vi "GroveSensors.vi"() -> ()   [LabVIEW 2016]
uses:
  VIs/uPythonX/uPythonX.xctl
panel:
  in  "Tab Control":enum32{"Button", "Pot", "Numbers"}(tab)=enum."Numbers"
  in  "Button":T1(xcontrol)={"VISA Refnum in"="ASRL23::INSTR", "Python Code"="import pyb,utime\n\nbutton = pyb.Pin('W16')\n\nbutton()\nutime.sleep(10)\nbutton()\n"}
  in  "Button 2":T1(xcontrol)={"VISA Refnum in"="ASRL23::INSTR", "Python Code"="import pyb,utime\n\nadc = pyb.ADC('W24')\n\nwhile True:\n     val = adc.read()\n     print ('%4.2f' % val)\n     utime.sleep_ms(200)\n     "}
  in  "Button 3":T1(xcontrol)={"VISA Refnum in"="ASRL23::INSTR", "Python Code"="import utime\n\ncharmap = {\n    '0': 0x3f,\n    '1': 0x06,\n    '2': 0x5b,\n    '3': 0x4f,\n    '4': 0x66,\n    '5': 0x6d,\n    '6': 0x7d,\n    '7': 0x07,\n    '8': 0x7f,\n    '9': 0x6f,\n    'A': 0x77,\n    'B': 0x7f,\n    'b': 0x7C,\n    'C': 0x39,\n    'c': 0x58,\n    'D': 0x3f,\n    'd': 0x5E,\n    'E': 0x79,\n    'F': 0x71,\n    'G': 0x7d,\n    'H': 0x76,\n    'h': 0x74,\n    'I': 0x06,\n    'J': 0x1f,\n    'K': 0x76,\n    'L': 0x38,\n    'l': 0x06,\n    'n': 0x54,\n    'O': 0x3f,\n    'o': 0x5c,\n    'P': 0x73,\n    'r': 0x50,\n    'S': 0x6d,\n    'U': 0x3e,\n    'V': 0x3e,\n    'Y': 0x66,\n    'Z': 0x5b,\n    '-': 0x40,\n    '_': 0x08,\n    ' ': 0x00\n}\n\nADDR_AUTO = 0x40\nADDR_FIXED = 0x44\nSTARTADDR = 0xC0\nBRIGHT_DARKEST = 0\nBRIGHT_DEFAULT = 2\nBRIGHT_HIGHEST = 7\n\nclass Grove4DigitDisplay(object):\n    colon_index = 1\n\n    def __init__(self, clk, dio, brightness=BRIGHT_DEFAULT):\n        self.brightness = brightness\n\n        self.clk = GPIO(clk, direction=GPIO.OUT)\n        self.dio = GPIO(dio, direction=GPIO.OUT)\n        self.data = [0] * 4\n        self.show_colon = False\n\n    def clear(self):\n        self.show_colon = False\n        self.data = [0] * 4\n        self._show()\n\n    def show(self, data):\n        if type(data) is str:\n            for i, c in enumerate(data):\n                if c in charmap:\n                    self.data[i] = charmap[c]\n                else:\n                    self.data[i] = 0\n                if i == self.colon_index and self.show_colon:\n                    self.data[i] |= 0x80\n                if i == 3:\n                    break\n        elif type(data) is int:\n            self.data = [0, 0, 0, charmap['0']]\n            if data < 0:\n                negative = True\n                data = -data\n            else:\n                negative = False\n            index = 3\n            while data != 0:\n                self.data[index] = charmap[str(data % 10)]\n                index -= 1\n                if index < 0:\n                    break\n                data = int(data / 10)\n\n            if negative:\n                if index >= 0:\n                    self.data[index] = charmap['-']\n                else:\n                    self.data = charmap['_'] + [charmap['9']] * 3\n        else:\n            raise ValueError('Not support {}'.format(type(data)))\n        self._show()\n\n    def _show(self):\n        with self:\n            self._transfer(ADDR_AUTO)\n\n        with self:\n            self._transfer(STARTADDR)\n            for i in range(4):\n                self._transfer(self.data[i])\n\n        with self:\n            self._transfer(0x88 + self.brightness)\n\n    def update(self, index, value):\n        if index < 0 or index > 4:\n            return\n\n        if value in charmap:\n            self.data[index] = charmap[value]\n        else:\n            self.data[index] = 0\n\n        if index == self.colon_index and self.show_colon:\n            self.data[index] |= 0x80\n\n        with self:\n            self._transfer(ADDR_FIXED)\n\n        with self:\n            self._transfer(STARTADDR | index)\n            self._transfer(self.data[index])\n\n        with self:\n            self._transfer(0x88 + self.brightness)\n\n\n    def set_brightness(self, brightness):\n        if brightness > 7:\n            brightness = 7\n\n        self.brightness = brightness\n        self._show()\n\n    def set_colon(self, enable):\n        self.show_colon = enable\n        if self.show_colon:\n            self.data[self.colon_index] |= 0x80\n        else:\n            self.data[self.colon_index] &= 0x7F\n        self._show()\n\n    def _transfer(self, data):\n        for _ in range(8):\n            self.clk.write(0)\n            if data & 0x01:\n                self.dio.write(1)\n            else:\n                self.dio.write(0)\n            data >>= 1\n            time.sleep(0.000001)\n            self.clk.write(1)\n            time.sleep(0.000001)\n\n        self.clk.write(0)\n        self.dio.write(1)\n        self.clk.write(1)\n        self.dio.dir(GPIO.IN)\n\n        while self.dio.read():\n            time.sleep(0.001)\n            if self.dio.read():\n                self.dio.dir(GPIO.OUT)\n                self.dio.write(0)\n                self.dio.dir(GPIO.IN)\n        self.dio.dir(GPIO.OUT)\n\n    def _start(self):\n        self.clk.write(1)\n        self.dio.write(1)\n        self.dio.write(0)\n        self.clk.write(0)\n\n    def _stop(self):\n        self.clk.write(0)\n        self.dio.write(0)\n        self.clk.write(1)\n        self.dio.write(1)\n\n    def __enter__(self):\n        self._start()\n\n    def __exit__(self, exc_type, exc_val, exc_tb):\n        self._stop()\n\ndisplay = Grove4DigitDisplay(clk = 'W16',dio = 'W22')\n\ncount = 0\nwhile True:\n     t = utime.strftime(\"%H%M\", time.localtime(time.time()))\n     display.show(t)\n     display.set_colon(count & 1)\n     count += 1\n     utime.sleep(1)\n"}
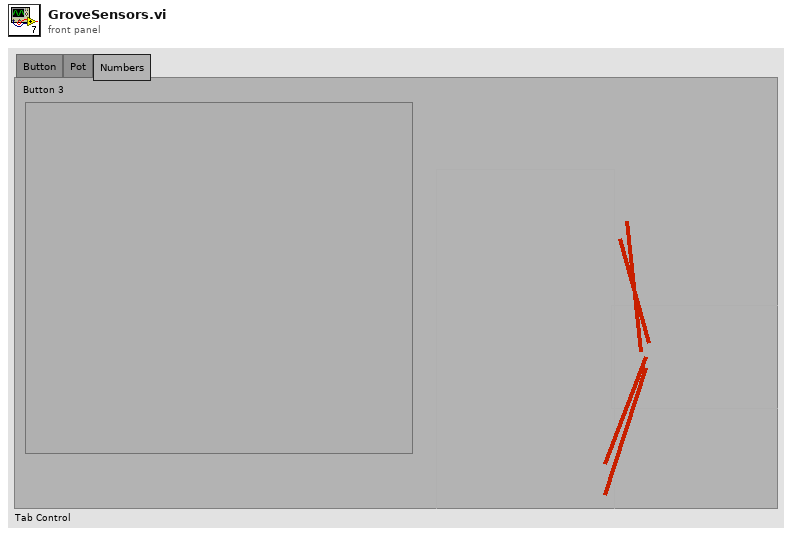
[diagram p1: front panel]
types:
  T1 = cluster{"VISA Refnum in":refnum<visa-resource-name>, "Python Code":string}
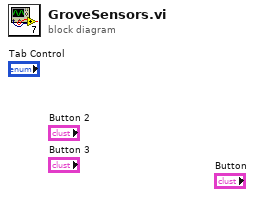
[diagram p0: block diagram]
diagram:
